vi "niRFSysCalReader EqvSetting Table Variant Name.vi"() -> (3 "Equivalent Setting Table Name":string)   [LabVIEW 2016, in "niRFSysCalReader.lvlib"]
uses:
  niRFSysCalReader.lvlib
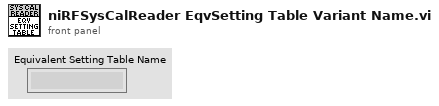
[diagram p1: front panel]
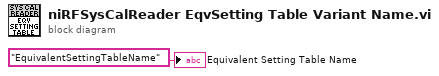
[diagram p0: block diagram]
diagram:
  "Equivalent Setting Table Name" <- "EquivalentSettingTableName" ("name")
